vi "Autonomous.vi"() -> ()   [LabVIEW 2023]
doc: "This VI starts when autonomous period begins, and will automatically be terminated when it ends. You can carry out timed or sensor driven operations directly to I/O or to subsystems without needing to return to the caller."
uses:
  <vilib>/Rock Robotics/WPI/Framework/Command Status Info.ctl
  <vilib>/Rock Robotics/WPI/Framework/Completion Status.ctl
  <vilib>/Rock Robotics/WPI/Framework/Completion Notifier.ctl
  Drive/Implementation/Drive Operations.ctl
  Support Code/Teleop Util/Coral States.ctl
  Support Code/Teleop Util/Scoring Levels.ctl
  Coral/Implementation/Coral Operations.ctl
  <vilib>/Rock Robotics/WPI/Utilities/WPI_GetSetVariantRefNum.vi
  Framework/Robot Global Data.vi
  <vilib>/Rock Robotics/Network Tables/NT Read String.vi
  <vilib>/Rock Robotics/Network Tables/NT Read String Array.vi
  <vilib>/Utility/file.llb/Read Delimited Spreadsheet (string).vi
panel:
  in  "Command Info Out 4":T1
  in  "Is Blue Alliance? 5":bool=TRUE
  in  "Command Info Out 3":T1
  in  "Is Blue Alliance? 4":bool=TRUE
  in  "Command Info Out 2":T1
  in  "Is Blue Alliance? 3":bool=TRUE
  in  "Command Info Out":T1
  in  "Is Blue Alliance? 2":bool=TRUE
  in  "Is Blue Alliance?":bool=TRUE
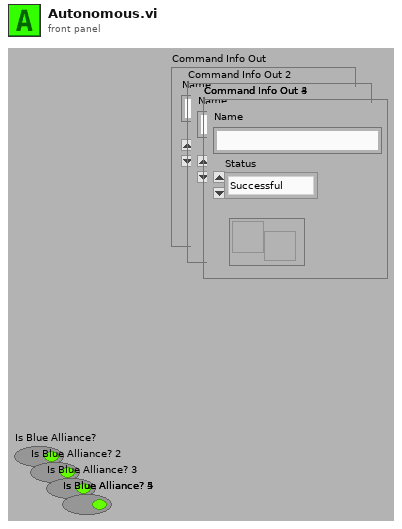
[diagram p1: front panel]
types:
  T1 = typedef "Command Status Info.ctl" = cluster{"Name":string, "Status":T2, "notifier out":T3}
  T2 = typedef "Completion Status.ctl" = enum16{"Successful", "Aborted", "Incomplete"}
  T3 = typedef "Completion Notifier.ctl" = refnum<notifier>
  T4 = typedef "WPI_JoystickDevRef.ctl" = cluster{"Device":T5}
  T5 = typedef "WPI_JoystickDeviceEnum.ctl" = enum16{"USB 0", "USB 1", "USB 2", "USB 3", "USB 4", "USB 5"}
  T6 = typedef "Drive Operations.ctl" = enum16{"Reserve", "Read Current", "Immediate", "Calibrate", "Reef Align", "Auto", "Old Reef Align"}
  T7 = typedef "Coral Operations.ctl" = enum16{"Reserve", "Read Current", "Immediate", "Calibrate"}
  T8 = typedef "Scoring Levels.ctl" = enum16{"Trough", "L2", "L3", "L4", "Default"}
  T9 = typedef "Coral States.ctl" = enum16{"Grounded", "Coral Intake", "Scoring Sequence", "Hold Position", "Score", "Manual Override", "Climb Safety Mode"}
  T10 = cluster{dbl, "Command out":cluster{"Name":string, "vi reference":refnum<vi>, i32[], variant[]}}[]
  T11 = typedef "Robot Velocities.ctl" = cluster{"X Velocity":dbl, "Y Velocity":dbl, "Rotational \nVelocity":dbl}
  T12 = typedef "CTRE_PigeonIMU_DeviceRef.ctl" = cluster{"DeviceStatus":errorcluster, "Device Number":u8, "Type":T13, "Device ID":u32, "Handle":u64, "UsageFrame":u32, "Library Path":path}
  T13 = typedef "CTRE_PigeonIMU_ConnectionType.ctl" = u32
  T14 = cluster{"Velocities":T11[], "Positions":cluster{"x":dbl, "y":dbl, "th":dbl}[], cluster{dbl, "Command out":cluster{"Name":string, "vi reference":refnum<vi>, i32[], variant[]}}[], "Zero Velocity?":bool[]}
  T15 = cluster{"Trough":dbl, "L2":dbl, "L3":dbl, "L4":dbl}
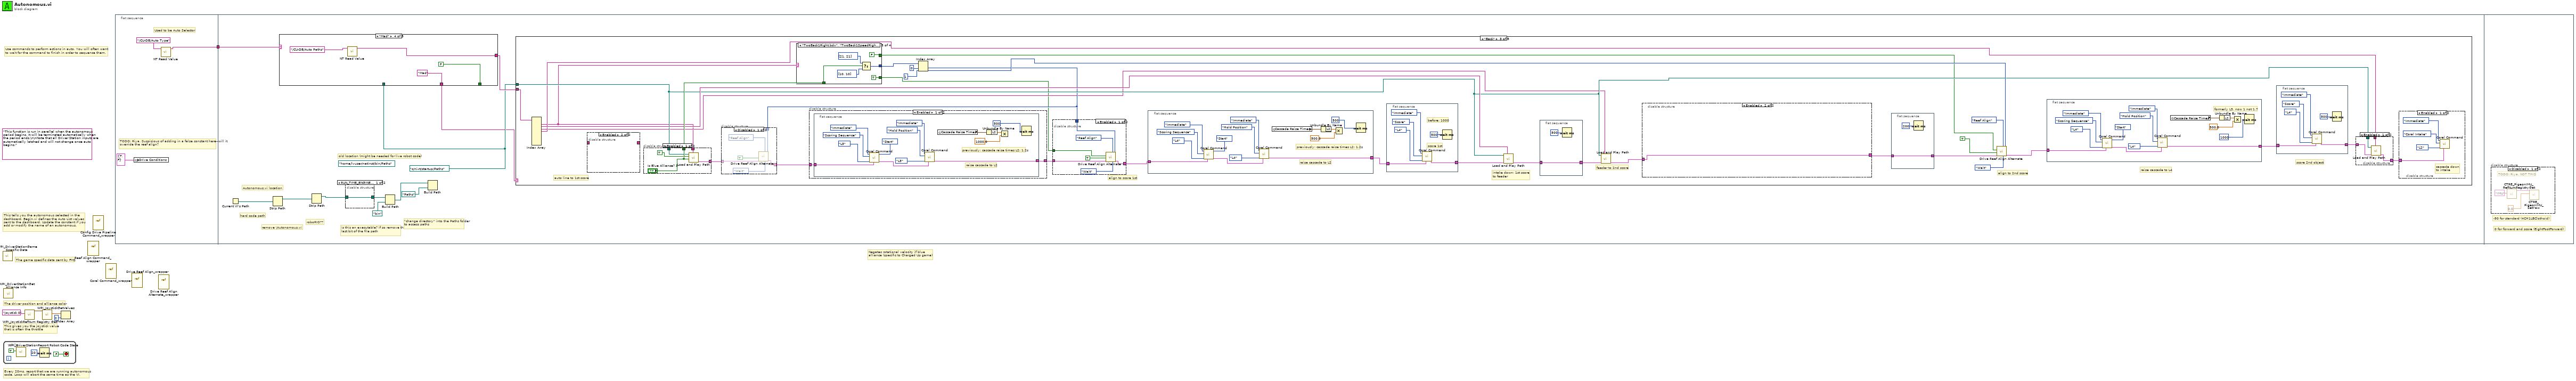
[diagram p0: block diagram]
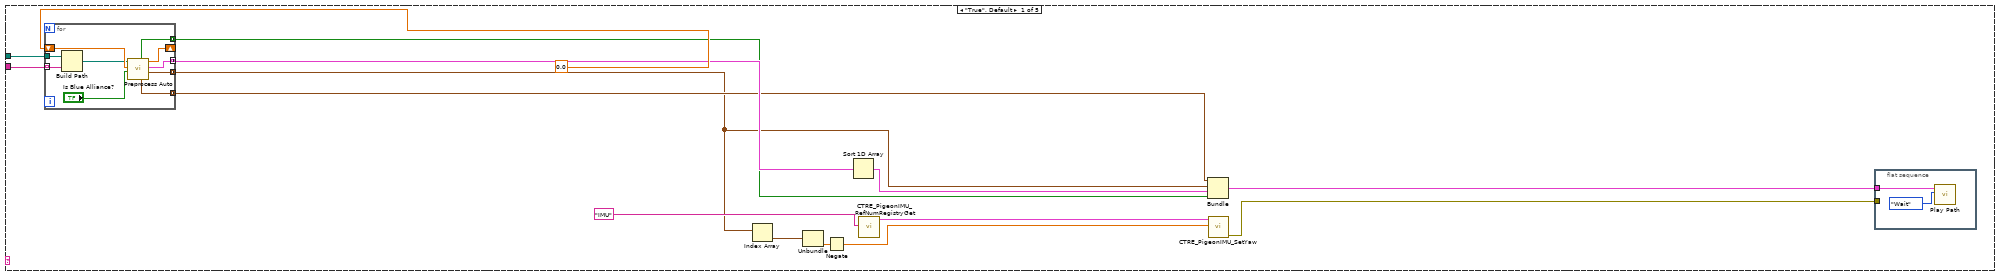
[diagram p2: hidden frame]
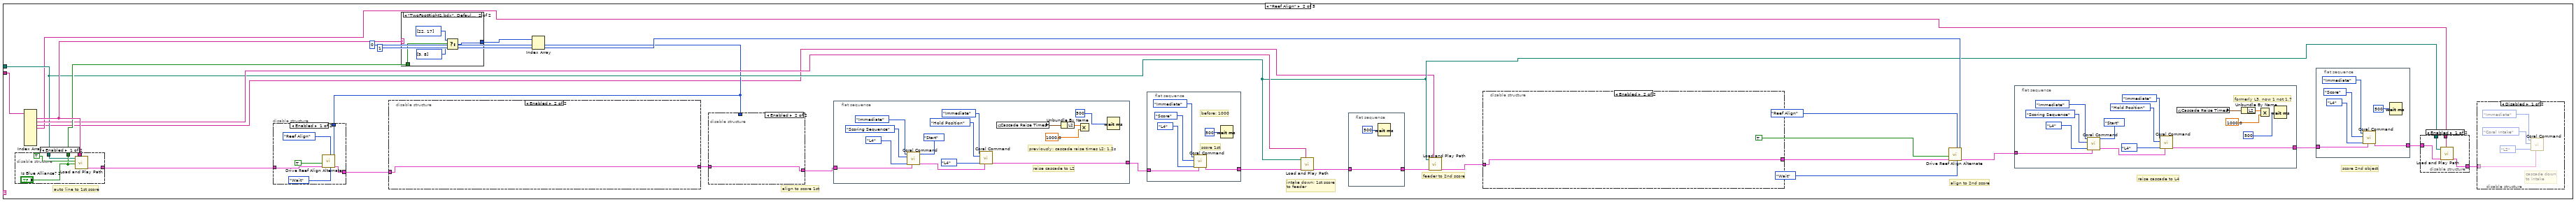
[diagram p3: hidden frame]
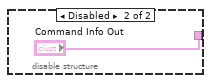
[diagram p4: hidden frame]
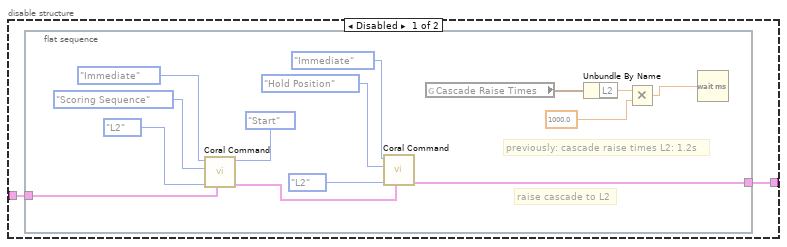
[diagram p6: hidden frame]
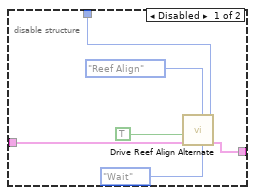
[diagram p8: hidden frame]
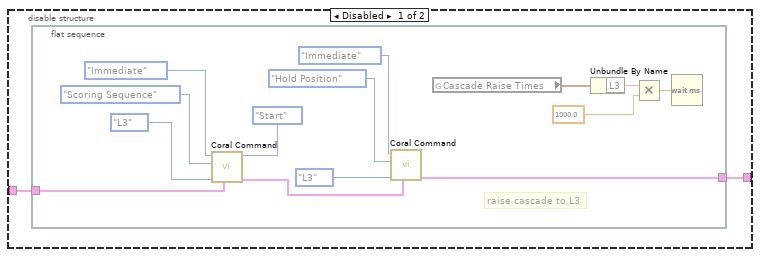
[diagram p9: hidden frame]
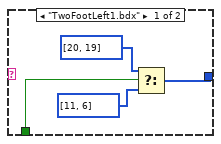
[diagram p11: hidden frame]
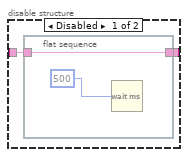
[diagram p12: hidden frame]
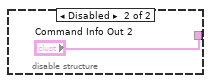
[diagram p13: hidden frame]
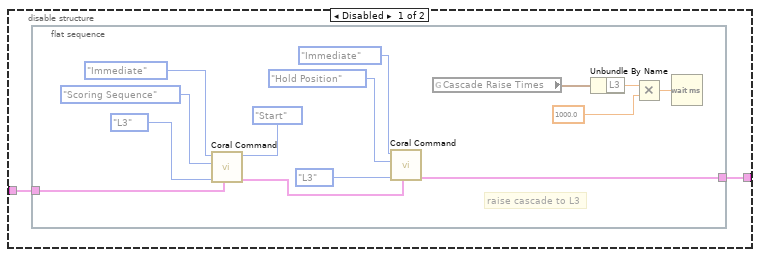
[diagram p18: hidden frame]
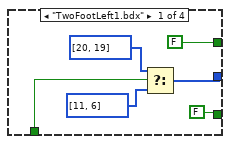
[diagram p20: hidden frame]
diagram:
  (unwired) "This function is run in parallel when the autonomous period begins. It will be terminated automatically when the period ends.\n\nNote that all Driver Station inputs are automatically latched and will not change once auto begins."
  # "Negates rotational velocity if blue alliance (specific to Charged Up game)"
  # "The game specific data sent by FMS"
  # "This tells you the autonomous selected in the \ndashboard. Begin.vi defines the Auto List values\nsent to the dashboard. Update the constant if you\nadd or modify the name of an autonomous."
  # "Every 20ms, report that we are running autonomous\ncode. Loop will abort the same time as the VI."
  # "This gives you the joystick value\nthat is often the throttle"
  # "Use commands to perform actions in auto. You will often want\nto wait for the command to finish in order to sequence them."
  # "The driver position and alliance color"
  n1 = call <vilib>:"WPI_DriverStationGame Specific Data.vi"() -> ()  [unwired: 11 in, 1 out]
  n2 = while {
    stop <- FALSE stop-if-true
    n3 = call <vilib>:"WPI_DriverStationReport Robot Code State.vi"("Autonomous"=TRUE) -> ()  [unwired: 10 in, 1 out]
    n4 = Wait (ms)(milliseconds to wait=u32 20) -> ()  [unwired: 1 out]
  }
  n5 = call <vilib>:"WPI_DriverStationGet Alliance Info.vi"() -> ()  [unwired: 12 out]
  n6 = call <vilib>:"WPI_JoystickRefNum Registry Get.vi"("refnum name"="Joystick 0") -> ("JoystickDevRef"=w4:T4)  [unwired: 1 in, 9 out]
  n7 = call <vilib>:"WPI_JoystickGetValues.vi"("JoystickDevRef"=w4) -> ("Axes"=w3:dbl[])  [unwired: 6 in, 4 out]
  n8 = Index Array(array=w3, index=2) -> ()  [unwired: 1 out]
  n9 = vi-ref "Reef Align Command_wrapper.vi"() -> ()  [unwired: 1 out]
  n10 = vi-ref "Config Drive Pipeline Command_wrapper.vi"() -> ()  [unwired: 1 out]
  n11 = vi-ref "Coral Command_wrapper.vi"() -> ()  [unwired: 1 out]
  n12 = flat-sequence {
    tunnel: [w9] -> w1
    tunnel: w1 -> [w13]
    frame #0 {
      # "Used to be Auto Selector"
      # "TODO: Riya. Suspicious of adding in a false constant here--will it override the reef align?"
      n13 = global write "Robot Global Data.vi" "Drive Conditions"(cluster{"Field Centric":bool, bool} {"Field Centric"=TRUE, FALSE} ("Drive Conditions")) -> ()
      n14 = call-poly <vilib>:"NT Read Value.vi"("name"="/CU-DB/Auto Type") -> ("value"=w9:string)  [unwired: 8 in, 2 out]
    }
    frame #1 {
      (unwired) path "/home/lvuser/natinst/bin/Paths"
      w14 = path "c:/ni-rt/startup/Paths"
      # "old location (might be needed for live robot code)"
      # "\"change directory\" into the Paths folder to access paths"
      # "is this an executable? if so remove that last bit of the file path"
      # "roboRIO??"
      # "remove \\Autonomous.vi"
      # "Autonomous.vi location"
      # "hard code path"
      n15 = Current VI's Path() -> (path=w19:path)
      n16 = Strip Path(path=w19) -> (stripped path=w20:path)  [unwired: 1 out]
      n17 = case shown="\"Mad\"" w13 {
        tunnel: w14 -> [_ _ _ _ w653]
        tunnel: [w631 w635 w639 w643 w647] -> w17
        tunnel: [TRUE FALSE FALSE FALSE TRUE ("Boolean")] -> _
        tunnel: ["" ("String") "Reef Align" "Back" "Mad" "" ("String")] -> w12
        frame "Manual", Default {
          n18 = call-poly <vilib>:"NT Read Value.vi"("name"="/CU-DB/Auto Paths") -> ("value"=w631:string[])  [unwired: 8 in, 2 out]
        }
        frame "Reef Align" {
          n19 = call-poly <vilib>:"NT Read Value.vi"("name"="/CU-DB/Auto Paths") -> ("value"=w635:string[])  [unwired: 8 in, 2 out]
        }
        frame "Back" {
          n20 = call-poly <vilib>:"NT Read Value.vi"("name"="/CU-DB/Auto Paths") -> ("value"=w639:string[])  [unwired: 8 in, 2 out]
        }
        frame "Mad" {
          n21 = call-poly <vilib>:"NT Read Value.vi"("name"="/CU-DB/Auto Paths") -> ("value"=w643:string[])  [unwired: 8 in, 2 out]
        }
        frame "Aquitaine" {
          n22 = call-poly <vilib>:"NT Read Value.vi"("name"="/CU-DB/Aquitaine") -> ("value"=w654:string)  [unwired: 8 in, 2 out]
          n23 = Build Path(base path=w653, name or relative path=w654) -> (appended path=w652:path)
          n24 = call-poly <vilib>:"Read Delimited Spreadsheet.vi"("file path (dialog if empty)"=w652) -> ("all rows"=w648:string[][])  [unwired: 9 in, 5 out]
          n25 = Array Size(array=w648) -> (size(s)=w651:i32[])
          n26 = Index Array(array=w651, index=0) -> (element=w649:i32)
          n27 = Reshape Array(w648, w649) -> (w647:string[])
        }
      }
      n28 = Strip Path(path=w20) -> (stripped path=w22:path)  [unwired: 1 out]
      n29 = disable-structure shown="RUN_TIME_ENGINE==False" {
        disable-tunnel: [w626 w627] -> w21
        disable-tunnel: w22 -> [w626 w628]
        frame condition #0 (active) {
        }
        frame condition #1 {
          n30 = Strip Path(path=w628) -> (stripped path=w627:path)  [unwired: 1 out]
        }
      }
      n31 = Build Path(base path=w21, name or relative path=path "bin") -> (appended path=w15:path)
      n32 = Build Path(base path=w15, name or relative path=path "Paths") -> ()  [unwired: 1 out]
      n33 = case shown="\"Back\"" w12 {
        tunnel: w17 -> [w26 w78 w223 w391 w539]
        tunnel: w14 -> [w25 w60 w207 w374 w531]
        frame "True", Default {
          n34 = for {
            tunnel: [w44] -> w28 mode=concatenating
            tunnel: [w45] -> w27 mode=concatenating
            shift-right: [w49] -> _
            shift-left: 0.0 -> [w47]
            tunnel: [w48] -> w34 mode=concatenating
            tunnel: [w43] -> w29 mode=concatenating
            tunnel: w25 -> [w40]
            tunnel: w26 -> [w41] mode=indexing
            n35 = Build Path(base path=w40, name or relative path=w41) -> (appended path=w42:path)
            n36 = call "Preprocess Auto.vi"("Is Blue Alliance?"="Is Blue Alliance?", "Start Time"=w47, "appended path"=w42) -> ("Positions"=w45:cluster{"x":dbl, "y":dbl, "th":dbl}[], "Array"=w48:T10, "Finish Time"=w49:dbl, "Velocities"=w44:T11[], "Zero Velocity?"=w43:bool[])  [unwired: 4 in]
          }
          n37 = Index Array(array=w27) -> (element=w33:cluster{"x":dbl, "y":dbl, "th":dbl})  [unwired: 1 in]
          n38 = Unbundle(w33) -> ("th"=w32:dbl)  [unwired: 2 out]
          n39 = Negate(x=w32) -> (-x=w31:dbl)
          n40 = Sort 1D Array(array=w34) -> (sorted array=w30:T10)
          n41 = call <vilib>:"CTRE_PigeonIMU_RefNumRegistryGet.vi"("refnum name"="IMU") -> ("PigeonIMUDevRef"=w37:T12)  [unwired: 9 in, 1 out]
          n42 = Bundle("Velocities"=w28, "Positions"=w27, w30, "Zero Velocity?"=w29) -> (w24:T14)  [unwired: 1 in]
          n43 = call <vilib>:"CTRE_PigeonIMU_SetYaw.vi"("Value"=w31, "PigeonIMUDevRef"=w37) -> ("error out"=w23:errorcluster)  [unwired: 8 in, 1 out]
          n44 = flat-sequence {
            tunnel: w24 -> [w38]
            tunnel: w23 -> [_]
            frame #0 {
              n45 = call "Play Path.vi"("Synchronization"=enum16{"Start", "Wait"}."Wait", "Auto Data"=w38) -> ()  [unwired: 9 in, 1 out]
            }
          }
        }
        frame "Reef Align" {
          # "score 2nd object"
          # "raise cascade to L4"
          # "align to 2nd score"
          # "feeder to 2nd score"
          # "intake down; 1st score\nto feeder"
          # "align to score 1st"
          # "auto line to 1st score"
          n46 = Index Array(array=w78) -> (element #1=w76:string, element #2=w72:string, element #3=w52:string, element #4=w59:string)  [unwired: 9 in, 5 out]
          n47 = disable-structure shown="Enabled" {
            disable-tunnel: w76 -> [w82 _]
            disable-tunnel: ["Is Blue Alliance? 2" _] -> w75
            disable-tunnel: w60 -> [w80 _]
            disable-tunnel: [w79 "Command Info Out"] -> w55
            frame Enabled {
              n48 = call "Load and Play Path.vi"("filename"=w82, "Is Blue Alliance? in"="Is Blue Alliance? 2", "Set IMU?"=TRUE, "Path"=w80) -> ("Command Info Out"=w79:T1)  [unwired: 6 in]
            }
            frame Disabled {
            }
          }
          n49 = case shown="\"TwoFootRight1.bdx\", Default" w76 {
            tunnel: w75 -> [w185 w189]
            tunnel: [w186 w188] -> w74
            frame "TwoFootLeft1.bdx" {
              n50 = Select(t=i32[] [20, 19], s=w185, f=i32[] [11, 6]) -> (s? t:f=w186:i32[])
            }
            frame "TwoFootRight1.bdx", Default {
              n51 = Select(t=i32[] [22, 17], s=w189, f=i32[] [9, 8]) -> (s? t:f=w188:i32[])
            }
          }
          n52 = Index Array(array=w74, index #1=0 ("index"), index #2=1 ("index")) -> (element #1=w53:i32, element #2=w63:i32)
          n53 = disable-structure shown="Enabled" {
            disable-tunnel: w55 -> [w122 w126]
            disable-tunnel: [w121 w126] -> w54
            disable-tunnel: w53 -> [w120 _]
            frame Enabled {
              n54 = call "Drive Reef Align Alternate.vi"("Tag ID"=w120, "Synchronication"=enum16{"Start", "Wait"}."Wait", "Operation"=Drive_Operations."Reef Align", "Command Info In"=w122, "Angle Align"=TRUE) -> ("Command Info Out"=w121:T1)  [unwired: 6 in]
            }
            frame Disabled {
            }
          }
          n55 = disable-structure shown="Enabled" {
            disable-tunnel: [w104 w119] -> w77
            disable-tunnel: w54 -> [w103 w119]
            frame Disabled {
              n56 = flat-sequence {
                tunnel: w103 -> [w118]
                tunnel: [w115] -> w104
                frame #0 {
                  # "previously: cascade raise times L2: 1.2s"
                  # "raise cascade to L2"
                  n57 = call "Coral Command.vi"("Synchronization"=enum16{"Start", "Wait"}."Start", "Command Info In"=w118, "Setpoint State"=Scoring_Levels."L2", "Coral States"=Coral_States."Scoring Sequence", "Operation"=Coral_Operations."Immediate") -> ("Command Info Out"=w116:T1)  [unwired: 5 in]
                  n58 = call "Coral Command.vi"("Command Info In"=w116, "Setpoint State"=Scoring_Levels."L2", "Coral States"=Coral_States."Hold Position", "Operation"=Coral_Operations."Immediate") -> ("Command Info Out"=w115:T1)  [unwired: 6 in]
                  n59 = global read "Robot Global Data.vi" "Cascade Raise Times"() -> (w108:T15)
                  n60 = Unbundle By Name(w108) -> ("L2"=w107:dbl)
                  n61 = Multiply(x=w107, y=1000.0) -> (x*y=w106:dbl)
                  n62 = Wait (ms)(milliseconds to wait=w106) -> ()  [unwired: 1 out]
                }
              }
            }
            frame Enabled {
            }
          }
          n63 = disable-structure shown="Enabled" {
            disable-tunnel: w77 -> [w132 w133]
            disable-tunnel: [w128 w133] -> w51
            disable-tunnel: w53 -> [w127 _]
            frame Disabled {
              n64 = call "Drive Reef Align Alternate.vi"("Tag ID"=w127, "Synchronication"=enum16{"Start", "Wait"}."Wait", "Operation"=Drive_Operations."Reef Align", "Command Info In"=w132, "Angle Align"=TRUE) -> ("Command Info Out"=w128:T1)  [unwired: 6 in]
            }
            frame Enabled {
            }
          }
          n65 = flat-sequence {
            tunnel: w51 -> [w102]
            tunnel: [w99] -> w50
            frame #0 {
              # "previously: cascade raise times L2: 1.2s"
              # "raise cascade to L2"
              n66 = call "Coral Command.vi"("Synchronization"=enum16{"Start", "Wait"}."Start", "Command Info In"=w102, "Setpoint State"=Scoring_Levels."L4", "Coral States"=Coral_States."Scoring Sequence", "Operation"=Coral_Operations."Immediate") -> ("Command Info Out"=w100:T1)  [unwired: 5 in]
              n67 = call "Coral Command.vi"("Command Info In"=w100, "Setpoint State"=Scoring_Levels."L4", "Coral States"=Coral_States."Hold Position", "Operation"=Coral_Operations."Immediate") -> ("Command Info Out"=w99:T1)  [unwired: 6 in]
              n68 = global read "Robot Global Data.vi" "Cascade Raise Times"() -> (w92:T15)
              n69 = Unbundle By Name(w92) -> ("L2"=w91:dbl)
              n70 = Multiply(x=w91, y=1000.0) -> ()  [unwired: 1 out]
              n71 = Wait (ms)(milliseconds to wait=u32 500) -> ()  [unwired: 1 out]
            }
          }
          n72 = flat-sequence {
            tunnel: w50 -> [w183]
            tunnel: [w178] -> w71
            frame #0 {
              # "before: 1000"
              # "score 1st"
              n73 = call "Coral Command.vi"("Command Info In"=w183, "Setpoint State"=Scoring_Levels."L4", "Coral States"=Coral_States."Score", "Operation"=Coral_Operations."Immediate") -> ("Command Info Out"=w178:T1)  [unwired: 6 in]
              n74 = Wait (ms)(milliseconds to wait=u32 500) -> ()  [unwired: 1 out]
            }
          }
          n75 = call "Load and Play Path.vi"("filename"=w72, "Command Info In"=w71, "Path"=w60) -> ("Command Info Out"=w70:T1)  [unwired: 7 in]
          n76 = flat-sequence {
            tunnel: w70 -> [w176]
            tunnel: [w176] -> w69
            frame #0 {
              n77 = Wait (ms)(milliseconds to wait=u32 500) -> ()  [unwired: 1 out]
            }
          }
          n78 = call "Load and Play Path.vi"("filename"=w52, "Command Info In"=w69, "Path"=w60) -> ("Command Info Out"=w68:T1)  [unwired: 7 in]
          n79 = disable-structure shown="Enabled" {
            disable-tunnel: w68 -> [w135 w150]
            disable-tunnel: [w134 w150] -> w66
            frame Disabled {
              n80 = flat-sequence {
                tunnel: w135 -> [w149]
                tunnel: [w146] -> w134
                frame #0 {
                  # "raise cascade to L3"
                  n81 = call "Coral Command.vi"("Synchronization"=enum16{"Start", "Wait"}."Start", "Command Info In"=w149, "Setpoint State"=Scoring_Levels."L3", "Coral States"=Coral_States."Scoring Sequence", "Operation"=Coral_Operations."Immediate") -> ("Command Info Out"=w147:T1)  [unwired: 5 in]
                  n82 = call "Coral Command.vi"("Command Info In"=w147, "Setpoint State"=Scoring_Levels."L3", "Coral States"=Coral_States."Hold Position", "Operation"=Coral_Operations."Immediate") -> ("Command Info Out"=w146:T1)  [unwired: 6 in]
                  n83 = global read "Robot Global Data.vi" "Cascade Raise Times"() -> (w139:T15)
                  n84 = Unbundle By Name(w139) -> ("L3"=w138:dbl)
                  n85 = Multiply(x=w138, y=1000.0) -> (x*y=w137:dbl)
                  n86 = Wait (ms)(milliseconds to wait=w137) -> ()  [unwired: 1 out]
                }
              }
            }
            frame Enabled {
            }
          }
          n87 = call "Drive Reef Align Alternate.vi"("Tag ID"=w63, "Synchronication"=enum16{"Start", "Wait"}."Wait", "Operation"=Drive_Operations."Reef Align", "Command Info In"=w66, "Angle Align"=TRUE) -> ("Command Info Out"=w57:T1)  [unwired: 6 in]
          n88 = flat-sequence {
            tunnel: w57 -> [w164]
            tunnel: [w161] -> w56
            frame #0 {
              # "formerly L3, now 1 not 1.7"
              n89 = call "Coral Command.vi"("Synchronization"=enum16{"Start", "Wait"}."Start", "Command Info In"=w164, "Setpoint State"=Scoring_Levels."L4", "Coral States"=Coral_States."Scoring Sequence", "Operation"=Coral_Operations."Immediate") -> ("Command Info Out"=w162:T1)  [unwired: 5 in]
              n90 = call "Coral Command.vi"("Command Info In"=w162, "Setpoint State"=Scoring_Levels."L4", "Coral States"=Coral_States."Hold Position", "Operation"=Coral_Operations."Immediate") -> ("Command Info Out"=w161:T1)  [unwired: 6 in]
              n91 = global read "Robot Global Data.vi" "Cascade Raise Times"() -> (w154:T15)
              n92 = Unbundle By Name(w154) -> ("L2"=w153:dbl)
              n93 = Multiply(x=w153, y=1000.0) -> ()  [unwired: 1 out]
              n94 = Wait (ms)(milliseconds to wait=u32 500) -> ()  [unwired: 1 out]
            }
          }
          n95 = flat-sequence {
            tunnel: w56 -> [w175]
            tunnel: [w170] -> w61
            frame #0 {
              n96 = call "Coral Command.vi"("Command Info In"=w175, "Setpoint State"=Scoring_Levels."L4", "Coral States"=Coral_States."Score", "Operation"=Coral_Operations."Immediate") -> ("Command Info Out"=w170:T1)  [unwired: 6 in]
              n97 = Wait (ms)(milliseconds to wait=u32 500) -> ()  [unwired: 1 out]
            }
          }
          n98 = disable-structure shown="Enabled" {
            disable-tunnel: w61 -> [w168 w169]
            disable-tunnel: w60 -> [w167 _]
            disable-tunnel: w59 -> [w166 _]
            disable-tunnel: [w165 w169] -> w58
            frame Enabled {
              n99 = call "Load and Play Path.vi"("filename"=w166, "Command Info In"=w168, "Path"=w167) -> ("Command Info Out"=w165:T1)  [unwired: 7 in]
            }
            frame Disabled {
            }
          }
          n100 = disable-structure shown="Disabled" {
            disable-tunnel: w58 -> [w85 _]
            frame Disabled {
              # "cascade down\nto intake"
              n101 = call "Coral Command.vi"("Command Info In"=w85, "Setpoint State"=Scoring_Levels."L2", "Coral States"=Coral_States."Coral Intake", "Operation"=Coral_Operations."Immediate") -> ()  [unwired: 6 in, 1 out]
            }
            frame Enabled {
            }
          }
        }
        frame "Back" {
          # "score 2nd object"
          # "raise cascade to L4"
          # "align to 2nd score"
          # "feeder to 2nd score"
          # "intake down; 1st score\nto feeder"
          # "align to score 1st"
          # "auto line to 1st score"
          n102 = Index Array(array=w223) -> (element #1=w192:string, element #2=w218:string, element #3=w199:string, element #4=w206:string)  [unwired: 9 in, 5 out]
          n103 = disable-structure shown="Enabled" {
            disable-tunnel: _ -> [w225 _]
            disable-tunnel: [w224 _] -> _
            frame Disabled {
              n104 = flat-sequence {
                tunnel: w225 -> [w227]
                tunnel: [w227] -> w224
                frame #0 {
                  n105 = Wait (ms)(milliseconds to wait=u32 500) -> ()  [unwired: 1 out]
                }
              }
            }
            frame Enabled {
            }
          }
          n106 = disable-structure shown="Enabled" {
            disable-tunnel: w192 -> [w233 _]
            disable-tunnel: ["Is Blue Alliance? 3" _] -> w221
            disable-tunnel: w207 -> [w231 _]
            disable-tunnel: [w230 "Command Info Out 2"] -> w202
            frame Enabled {
              n107 = call "Load and Play Path.vi"("filename"=w233, "Is Blue Alliance? in"="Is Blue Alliance? 3", "Set IMU?"=TRUE, "Path"=w231) -> ("Command Info Out"=w230:T1)  [unwired: 6 in]
            }
            frame Disabled {
            }
          }
          n108 = case shown="\"TwoBack1Right.bdx\", \"TwoBack1SpeedRight.bdx\"" w192 {
            tunnel: w221 -> [w339 w345 w351 w357]
            tunnel: [w340 w344 w350 w356] -> w220
            tunnel: [FALSE FALSE TRUE FALSE] -> w194
            tunnel: [FALSE TRUE FALSE FALSE] -> w193
            frame "TwoFootLeft1.bdx" {
              n109 = Select(t=i32[] [20, 19], s=w339, f=i32[] [11, 6]) -> (s? t:f=w340:i32[])
            }
            frame "TwoBack1.bdx", "TwoBack1Speed.bdx", Default {
              n110 = Select(t=i32[] [21, 21], s=w345, f=i32[] [10, 10]) -> (s? t:f=w344:i32[])
            }
            frame "TwoBack1Right.bdx", "TwoBack1SpeedRight.bdx" {
              n111 = Select(t=i32[] [21, 21], s=w351, f=i32[] [10, 10]) -> (s? t:f=w350:i32[])
            }
            frame "TwoFootRight1.bdx" {
              n112 = Select(t=i32[] [22, 17], s=w357, f=i32[] [9, 8]) -> (s? t:f=w356:i32[])
            }
          }
          n113 = Index Array(array=w220, index #1=0 ("index"), index #2=1 ("index")) -> (element #1=w200:i32, element #2=w210:i32)
          n114 = disable-structure shown="Disabled" {
            disable-tunnel: w202 -> [w273 w277]
            disable-tunnel: [w272 w277] -> w201
            disable-tunnel: w200 -> [w271 _]
            frame Disabled {
              n115 = call "Drive Reef Align Alternate.vi"("Tag ID"=w271, "Synchronication"=enum16{"Start", "Wait"}."Wait", "Operation"=Drive_Operations."Reef Align", "Command Info In"=w273, "Angle Align"=TRUE) -> ("Command Info Out"=w272:T1)  [unwired: 6 in]
            }
            frame Enabled {
            }
          }
          n116 = disable-structure shown="Enabled" {
            disable-tunnel: [w255 w270] -> w222
            disable-tunnel: w201 -> [w254 w270]
            frame Enabled {
              n117 = flat-sequence {
                tunnel: w254 -> [w269]
                tunnel: [w266] -> w255
                frame #0 {
                  # "previously: cascade raise times L2: 1.2s"
                  # "raise cascade to L2"
                  n118 = call "Coral Command.vi"("Synchronization"=enum16{"Start", "Wait"}."Start", "Command Info In"=w269, "Setpoint State"=Scoring_Levels."L3", "Coral States"=Coral_States."Scoring Sequence", "Operation"=Coral_Operations."Immediate") -> ("Command Info Out"=w267:T1)  [unwired: 5 in]
                  n119 = call "Coral Command.vi"("Command Info In"=w267, "Setpoint State"=Scoring_Levels."L3", "Coral States"=Coral_States."Hold Position", "Operation"=Coral_Operations."Immediate") -> ("Command Info Out"=w266:T1)  [unwired: 6 in]
                  n120 = global read "Robot Global Data.vi" "Cascade Raise Times"() -> (w259:T15)
                  n121 = Unbundle By Name(w259) -> ("L2"=w258:dbl)
                  n122 = Multiply(x=w258, y=1000.0) -> ()  [unwired: 1 out]
                  n123 = Wait (ms)(milliseconds to wait=u32 500) -> ()  [unwired: 1 out]
                }
              }
            }
            frame Disabled {
            }
          }
          n124 = disable-structure shown="Enabled" {
            disable-tunnel: w222 -> [w284 w285]
            disable-tunnel: [w280 w285] -> w198
            disable-tunnel: w200 -> [w279 _]
            disable-tunnel: w194 -> [w278 _]
            frame Enabled {
              n125 = call "Drive Reef Align Alternate.vi"("Tag ID"=w279, "Synchronication"=enum16{"Start", "Wait"}."Wait", "Operation"=Drive_Operations."Reef Align", "Command Info In"=w284, "Angle Align"=TRUE, "Left side"=w278) -> ("Command Info Out"=w280:T1)  [unwired: 5 in]
            }
            frame Disabled {
            }
          }
          n126 = flat-sequence {
            tunnel: w198 -> [w253]
            tunnel: [w250] -> w197
            frame #0 {
              # "previously: cascade raise times L2: 1.2s"
              # "raise cascade to L2"
              n127 = call "Coral Command.vi"("Synchronization"=enum16{"Start", "Wait"}."Start", "Command Info In"=w253, "Setpoint State"=Scoring_Levels."L4", "Coral States"=Coral_States."Scoring Sequence", "Operation"=Coral_Operations."Immediate") -> ("Command Info Out"=w251:T1)  [unwired: 5 in]
              n128 = call "Coral Command.vi"("Command Info In"=w251, "Setpoint State"=Scoring_Levels."L4", "Coral States"=Coral_States."Hold Position", "Operation"=Coral_Operations."Immediate") -> ("Command Info Out"=w250:T1)  [unwired: 6 in]
              n129 = global read "Robot Global Data.vi" "Cascade Raise Times"() -> (w243:T15)
              n130 = Unbundle By Name(w243) -> ("L2"=w242:dbl)
              n131 = Multiply(x=w242, y=500.0) -> ()  [unwired: 1 out]
              n132 = Wait (ms)(milliseconds to wait=u32 500) -> ()  [unwired: 1 out]
            }
          }
          n133 = flat-sequence {
            tunnel: w197 -> [w335]
            tunnel: [w330] -> w217
            frame #0 {
              # "before: 1000"
              # "score 1st"
              n134 = call "Coral Command.vi"("Command Info In"=w335, "Setpoint State"=Scoring_Levels."L4", "Coral States"=Coral_States."Score", "Operation"=Coral_Operations."Immediate") -> ("Command Info Out"=w330:T1)  [unwired: 6 in]
              n135 = Wait (ms)(milliseconds to wait=u32 500) -> ()  [unwired: 1 out]
            }
          }
          n136 = call "Load and Play Path.vi"("filename"=w218, "Command Info In"=w217, "Path"=w207) -> ("Command Info Out"=w216:T1)  [unwired: 7 in]
          n137 = flat-sequence {
            tunnel: w216 -> [w328]
            tunnel: [w328] -> w215
            frame #0 {
              n138 = Wait (ms)(milliseconds to wait=u32 500) -> ()  [unwired: 1 out]
            }
          }
          n139 = call "Load and Play Path.vi"("filename"=w199, "Command Info In"=w215, "Path"=w207) -> ("Command Info Out"=w214:T1)  [unwired: 7 in]
          n140 = disable-structure shown="Enabled" {
            disable-tunnel: w214 -> [w287 w302]
            disable-tunnel: [w286 w302] -> w196
            frame Disabled {
              n141 = flat-sequence {
                tunnel: w287 -> [w301]
                tunnel: [w298] -> w286
                frame #0 {
                  # "raise cascade to L3"
                  n142 = call "Coral Command.vi"("Synchronization"=enum16{"Start", "Wait"}."Start", "Command Info In"=w301, "Setpoint State"=Scoring_Levels."L3", "Coral States"=Coral_States."Scoring Sequence", "Operation"=Coral_Operations."Immediate") -> ("Command Info Out"=w299:T1)  [unwired: 5 in]
                  n143 = call "Coral Command.vi"("Command Info In"=w299, "Setpoint State"=Scoring_Levels."L3", "Coral States"=Coral_States."Hold Position", "Operation"=Coral_Operations."Immediate") -> ("Command Info Out"=w298:T1)  [unwired: 6 in]
                  n144 = global read "Robot Global Data.vi" "Cascade Raise Times"() -> (w291:T15)
                  n145 = Unbundle By Name(w291) -> ("L3"=w290:dbl)
                  n146 = Multiply(x=w290, y=1000.0) -> (x*y=w289:dbl)
                  n147 = Wait (ms)(milliseconds to wait=w289) -> ()  [unwired: 1 out]
                }
              }
            }
            frame Enabled {
            }
          }
          n148 = flat-sequence {
            tunnel: w196 -> [w228]
            tunnel: [w228] -> w195
            frame #0 {
              n149 = Wait (ms)(milliseconds to wait=u32 200) -> ()  [unwired: 1 out]
            }
          }
          n150 = call "Drive Reef Align Alternate.vi"("Tag ID"=w210, "Synchronication"=enum16{"Start", "Wait"}."Wait", "Operation"=Drive_Operations."Reef Align", "Command Info In"=w195, "Angle Align"=TRUE, "Left side"=w193) -> ("Command Info Out"=w204:T1)  [unwired: 5 in]
          n151 = flat-sequence {
            tunnel: w204 -> [w316]
            tunnel: [w313] -> w203
            frame #0 {
              # "formerly L3, now 1 not 1.7"
              n152 = call "Coral Command.vi"("Synchronization"=enum16{"Start", "Wait"}."Start", "Command Info In"=w316, "Setpoint State"=Scoring_Levels."L4", "Coral States"=Coral_States."Scoring Sequence", "Operation"=Coral_Operations."Immediate") -> ("Command Info Out"=w314:T1)  [unwired: 5 in]
              n153 = call "Coral Command.vi"("Command Info In"=w314, "Setpoint State"=Scoring_Levels."L4", "Coral States"=Coral_States."Hold Position", "Operation"=Coral_Operations."Immediate") -> ("Command Info Out"=w313:T1)  [unwired: 6 in]
              n154 = global read "Robot Global Data.vi" "Cascade Raise Times"() -> (w306:T15)
              n155 = Unbundle By Name(w306) -> ("L2"=w305:dbl)
              n156 = Multiply(x=w305, y=500.0) -> ()  [unwired: 1 out]
              n157 = Wait (ms)(milliseconds to wait=u32 1000) -> ()  [unwired: 1 out]
            }
          }
          n158 = flat-sequence {
            tunnel: w203 -> [w327]
            tunnel: [w322] -> w208
            frame #0 {
              n159 = call "Coral Command.vi"("Command Info In"=w327, "Setpoint State"=Scoring_Levels."L4", "Coral States"=Coral_States."Score", "Operation"=Coral_Operations."Immediate") -> ("Command Info Out"=w322:T1)  [unwired: 6 in]
              n160 = Wait (ms)(milliseconds to wait=u32 500) -> ()  [unwired: 1 out]
            }
          }
          n161 = disable-structure shown="Enabled" {
            disable-tunnel: w208 -> [w320 w321]
            disable-tunnel: w207 -> [w319 _]
            disable-tunnel: w206 -> [w318 _]
            disable-tunnel: [w317 w321] -> w205
            frame Enabled {
              n162 = call "Load and Play Path.vi"("filename"=w318, "Command Info In"=w320, "Path"=w319) -> ("Command Info Out"=w317:T1)  [unwired: 7 in]
            }
            frame Disabled {
            }
          }
          n163 = disable-structure shown="Enabled" {
            disable-tunnel: w205 -> [w236 _]
            frame Enabled {
              # "cascade down\nto intake"
              n164 = call "Coral Command.vi"("Command Info In"=w236, "Setpoint State"=Scoring_Levels."L2", "Coral States"=Coral_States."Coral Intake", "Operation"=Coral_Operations."Immediate") -> ()  [unwired: 6 in, 1 out]
            }
            frame Disabled {
            }
          }
        }
        frame "Mad" {
          # "score 2nd object"
          # "raise cascade to L4"
          # "align to 2nd score"
          # "feeder to 2nd score"
          # "intake down; 1st score\nto feeder"
          # "align to score 1st"
          # "auto line to 1st score"
          n165 = Index Array(array=w391) -> (element #1=w389:string, element #2=w385:string, element #3=w366:string, element #4=w373:string)  [unwired: 9 in, 5 out]
          n166 = disable-structure shown="Enabled" {
            disable-tunnel: w389 -> [w397 _]
            disable-tunnel: ["Is Blue Alliance? 5" _] -> w388
            disable-tunnel: w374 -> [w395 _]
            disable-tunnel: [w394 "Command Info Out 4"] -> w369
            frame Enabled {
              n167 = call "Load and Play Path.vi"("filename"=w397, "Is Blue Alliance? in"="Is Blue Alliance? 5", "Set IMU?"=TRUE, "Path"=w395) -> ("Command Info Out"=w394:T1)  [unwired: 6 in]
            }
            frame Disabled {
            }
          }
          n168 = case shown="\"TwoBack1Right.bdx\", \"TwoBack1SpeedRight.bdx\"" w389 {
            tunnel: w388 -> [w503 w509 w515 w521]
            tunnel: [w504 w508 w514 w520] -> w387
            tunnel: [FALSE FALSE TRUE FALSE] -> w361
            tunnel: [FALSE TRUE FALSE FALSE] -> w360
            frame "TwoFootLeft1.bdx" {
              n169 = Select(t=i32[] [20, 19], s=w503, f=i32[] [11, 6]) -> (s? t:f=w504:i32[])
            }
            frame "TwoBack1.bdx", "TwoBack1Speed.bdx", Default {
              n170 = Select(t=i32[] [21, 19], s=w509, f=i32[] [10, 6]) -> (s? t:f=w508:i32[])
            }
            frame "TwoBack1Right.bdx", "TwoBack1SpeedRight.bdx" {
              n171 = Select(t=i32[] [21, 17], s=w515, f=i32[] [10, 8]) -> (s? t:f=w514:i32[])
            }
            frame "TwoFootRight1.bdx" {
              n172 = Select(t=i32[] [22, 17], s=w521, f=i32[] [9, 8]) -> (s? t:f=w520:i32[])
            }
          }
          n173 = Index Array(array=w387, index #1=0 ("index"), index #2=1 ("index")) -> (element #1=w367:i32, element #2=w377:i32)
          n174 = disable-structure shown="Disabled" {
            disable-tunnel: w369 -> [w437 w441]
            disable-tunnel: [w436 w441] -> w368
            disable-tunnel: w367 -> [w435 _]
            frame Disabled {
              n175 = call "Drive Reef Align Alternate.vi"("Tag ID"=w435, "Synchronication"=enum16{"Start", "Wait"}."Wait", "Operation"=Drive_Operations."Reef Align", "Command Info In"=w437, "Angle Align"=TRUE) -> ("Command Info Out"=w436:T1)  [unwired: 6 in]
            }
            frame Enabled {
            }
          }
          n176 = disable-structure shown="Enabled" {
            disable-tunnel: [w419 w434] -> w390
            disable-tunnel: w368 -> [w418 w434]
            frame Enabled {
              n177 = flat-sequence {
                tunnel: w418 -> [w433]
                tunnel: [w430] -> w419
                frame #0 {
                  # "previously: cascade raise times L2: 1.2s"
                  # "raise cascade to L2"
                  n178 = call "Coral Command.vi"("Synchronization"=enum16{"Start", "Wait"}."Start", "Command Info In"=w433, "Setpoint State"=Scoring_Levels."L3", "Coral States"=Coral_States."Scoring Sequence", "Operation"=Coral_Operations."Immediate") -> ("Command Info Out"=w431:T1)  [unwired: 5 in]
                  n179 = call "Coral Command.vi"("Command Info In"=w431, "Setpoint State"=Scoring_Levels."L3", "Coral States"=Coral_States."Hold Position", "Operation"=Coral_Operations."Immediate") -> ("Command Info Out"=w430:T1)  [unwired: 6 in]
                  n180 = global read "Robot Global Data.vi" "Cascade Raise Times"() -> (w423:T15)
                  n181 = Unbundle By Name(w423) -> ("L2"=w422:dbl)
                  n182 = Multiply(x=w422, y=1000.0) -> ()  [unwired: 1 out]
                  n183 = Wait (ms)(milliseconds to wait=u32 500) -> ()  [unwired: 1 out]
                }
              }
            }
            frame Disabled {
            }
          }
          n184 = disable-structure shown="Enabled" {
            disable-tunnel: w390 -> [w448 w449]
            disable-tunnel: [w444 w449] -> w365
            disable-tunnel: w367 -> [w443 _]
            disable-tunnel: w361 -> [w442 _]
            frame Enabled {
              n185 = call "Drive Reef Align Alternate.vi"("Tag ID"=w443, "Synchronication"=enum16{"Start", "Wait"}."Wait", "Operation"=Drive_Operations."Reef Align", "Command Info In"=w448, "Angle Align"=TRUE, "Left side"=w442) -> ("Command Info Out"=w444:T1)  [unwired: 5 in]
            }
            frame Disabled {
            }
          }
          n186 = flat-sequence {
            tunnel: w365 -> [w417]
            tunnel: [w414] -> w364
            frame #0 {
              # "previously: cascade raise times L2: 1.2s"
              # "raise cascade to L2"
              n187 = call "Coral Command.vi"("Synchronization"=enum16{"Start", "Wait"}."Start", "Command Info In"=w417, "Setpoint State"=Scoring_Levels."L4", "Coral States"=Coral_States."Scoring Sequence", "Operation"=Coral_Operations."Immediate") -> ("Command Info Out"=w415:T1)  [unwired: 5 in]
              n188 = call "Coral Command.vi"("Command Info In"=w415, "Setpoint State"=Scoring_Levels."L4", "Coral States"=Coral_States."Hold Position", "Operation"=Coral_Operations."Immediate") -> ("Command Info Out"=w414:T1)  [unwired: 6 in]
              n189 = global read "Robot Global Data.vi" "Cascade Raise Times"() -> (w407:T15)
              n190 = Unbundle By Name(w407) -> ("L2"=w406:dbl)
              n191 = Multiply(x=w406, y=500.0) -> ()  [unwired: 1 out]
              n192 = Wait (ms)(milliseconds to wait=u32 500) -> ()  [unwired: 1 out]
            }
          }
          n193 = flat-sequence {
            tunnel: w364 -> [w499]
            tunnel: [w494] -> w384
            frame #0 {
              # "before: 1000"
              # "score 1st"
              n194 = call "Coral Command.vi"("Command Info In"=w499, "Setpoint State"=Scoring_Levels."L4", "Coral States"=Coral_States."Score", "Operation"=Coral_Operations."Immediate") -> ("Command Info Out"=w494:T1)  [unwired: 6 in]
              n195 = Wait (ms)(milliseconds to wait=u32 500) -> ()  [unwired: 1 out]
            }
          }
          n196 = call "Load and Play Path.vi"("filename"=w385, "Command Info In"=w384, "Path"=w374) -> ("Command Info Out"=w383:T1)  [unwired: 7 in]
          n197 = flat-sequence {
            tunnel: w383 -> [w492]
            tunnel: [w492] -> w382
            frame #0 {
              n198 = Wait (ms)(milliseconds to wait=u32 500) -> ()  [unwired: 1 out]
            }
          }
          n199 = call "Load and Play Path.vi"("filename"=w366, "Command Info In"=w382, "Path"=w374) -> ("Command Info Out"=w381:T1)  [unwired: 7 in]
          n200 = disable-structure shown="Enabled" {
            disable-tunnel: w381 -> [w451 w466]
            disable-tunnel: [w450 w466] -> w363
            frame Disabled {
              n201 = flat-sequence {
                tunnel: w451 -> [w465]
                tunnel: [w462] -> w450
                frame #0 {
                  # "raise cascade to L3"
                  n202 = call "Coral Command.vi"("Synchronization"=enum16{"Start", "Wait"}."Start", "Command Info In"=w465, "Setpoint State"=Scoring_Levels."L3", "Coral States"=Coral_States."Scoring Sequence", "Operation"=Coral_Operations."Immediate") -> ("Command Info Out"=w463:T1)  [unwired: 5 in]
                  n203 = call "Coral Command.vi"("Command Info In"=w463, "Setpoint State"=Scoring_Levels."L3", "Coral States"=Coral_States."Hold Position", "Operation"=Coral_Operations."Immediate") -> ("Command Info Out"=w462:T1)  [unwired: 6 in]
                  n204 = global read "Robot Global Data.vi" "Cascade Raise Times"() -> (w455:T15)
                  n205 = Unbundle By Name(w455) -> ("L3"=w454:dbl)
                  n206 = Multiply(x=w454, y=1000.0) -> (x*y=w453:dbl)
                  n207 = Wait (ms)(milliseconds to wait=w453) -> ()  [unwired: 1 out]
                }
              }
            }
            frame Enabled {
            }
          }
          n208 = flat-sequence {
            tunnel: w363 -> [w392]
            tunnel: [w392] -> w362
            frame #0 {
              n209 = Wait (ms)(milliseconds to wait=u32 200) -> ()  [unwired: 1 out]
            }
          }
          n210 = call "Drive Reef Align Alternate.vi"("Tag ID"=w377, "Synchronication"=enum16{"Start", "Wait"}."Wait", "Operation"=Drive_Operations."Reef Align", "Command Info In"=w362, "Angle Align"=TRUE, "Left side"=w360) -> ("Command Info Out"=w371:T1)  [unwired: 5 in]
          n211 = flat-sequence {
            tunnel: w371 -> [w480]
            tunnel: [w477] -> w370
            frame #0 {
              # "formerly L3, now 1 not 1.7"
              n212 = call "Coral Command.vi"("Synchronization"=enum16{"Start", "Wait"}."Start", "Command Info In"=w480, "Setpoint State"=Scoring_Levels."L4", "Coral States"=Coral_States."Scoring Sequence", "Operation"=Coral_Operations."Immediate") -> ("Command Info Out"=w478:T1)  [unwired: 5 in]
              n213 = call "Coral Command.vi"("Command Info In"=w478, "Setpoint State"=Scoring_Levels."L4", "Coral States"=Coral_States."Hold Position", "Operation"=Coral_Operations."Immediate") -> ("Command Info Out"=w477:T1)  [unwired: 6 in]
              n214 = global read "Robot Global Data.vi" "Cascade Raise Times"() -> (w470:T15)
              n215 = Unbundle By Name(w470) -> ("L2"=w469:dbl)
              n216 = Multiply(x=w469, y=500.0) -> ()  [unwired: 1 out]
              n217 = Wait (ms)(milliseconds to wait=u32 1000) -> ()  [unwired: 1 out]
            }
          }
          n218 = flat-sequence {
            tunnel: w370 -> [w491]
            tunnel: [w486] -> w375
            frame #0 {
              n219 = call "Coral Command.vi"("Command Info In"=w491, "Setpoint State"=Scoring_Levels."L4", "Coral States"=Coral_States."Score", "Operation"=Coral_Operations."Immediate") -> ("Command Info Out"=w486:T1)  [unwired: 6 in]
              n220 = Wait (ms)(milliseconds to wait=u32 500) -> ()  [unwired: 1 out]
            }
          }
          n221 = disable-structure shown="Enabled" {
            disable-tunnel: w375 -> [w484 w485]
            disable-tunnel: w374 -> [w483 _]
            disable-tunnel: w373 -> [w482 _]
            disable-tunnel: [w481 w485] -> w372
            frame Enabled {
              n222 = call "Load and Play Path.vi"("filename"=w482, "Command Info In"=w484, "Path"=w483) -> ("Command Info Out"=w481:T1)  [unwired: 7 in]
            }
            frame Disabled {
            }
          }
          n223 = disable-structure shown="Enabled" {
            disable-tunnel: w372 -> [w400 _]
            frame Enabled {
              # "cascade down\nto intake"
              n224 = call "Coral Command.vi"("Command Info In"=w400, "Setpoint State"=Scoring_Levels."L2", "Coral States"=Coral_States."Coral Intake", "Operation"=Coral_Operations."Immediate") -> ()  [unwired: 6 in, 1 out]
            }
            frame Disabled {
            }
          }
        }
        frame "Short Back" {
          # "align to score 1st"
          # "auto line to 1st score"
          n225 = Index Array(array=w539) -> (element #1=w537:string, element #2=w533:string)  [unwired: 9 in, 7 out]
          n226 = disable-structure shown="Enabled" {
            disable-tunnel: w537 -> [w547 _]
            disable-tunnel: ["Is Blue Alliance? 4" _] -> w536
            disable-tunnel: w531 -> [w545 _]
            disable-tunnel: [w544 "Command Info Out 3"] -> w530
            frame Enabled {
              n227 = call "Load and Play Path.vi"("filename"=w547, "Is Blue Alliance? in"="Is Blue Alliance? 4", "Set IMU?"=TRUE, "Path"=w545) -> ("Command Info Out"=w544:T1)  [unwired: 6 in]
            }
            frame Disabled {
            }
          }
          n228 = case shown="\"TwoBack1Right.bdx\", \"TwoBack1SpeedRight.bdx\"" w537 {
            tunnel: w536 -> [w605 w611 w617 w623]
            tunnel: [w606 w610 w616 w622] -> w535
            tunnel: [FALSE FALSE TRUE FALSE] -> w525
            tunnel: [FALSE TRUE FALSE FALSE] -> _
            frame "TwoFootLeft1.bdx" {
              n229 = Select(t=i32[] [20, 19], s=w605, f=i32[] [11, 6]) -> (s? t:f=w606:i32[])
            }
            frame "TwoBack1.bdx", "TwoBack1Speed.bdx" {
              n230 = Select(t=i32[] [21, 21], s=w611, f=i32[] [10, 10]) -> (s? t:f=w610:i32[])
            }
            frame "TwoBack1Right.bdx", "TwoBack1SpeedRight.bdx" {
              n231 = Select(t=i32[] [21, 21], s=w617, f=i32[] [10, 10]) -> (s? t:f=w616:i32[])
            }
            frame "TwoFootRight1.bdx", Default {
              n232 = Select(t=i32[] [22, 17], s=w623, f=i32[] [9, 8]) -> (s? t:f=w622:i32[])
            }
          }
          n233 = Index Array(array=w535, index=0) -> (element=w528:i32)
          n234 = disable-structure shown="Disabled" {
            disable-tunnel: w530 -> [w583 w587]
            disable-tunnel: [w582 w587] -> w529
            disable-tunnel: w528 -> [w581 _]
            frame Disabled {
              n235 = call "Drive Reef Align Alternate.vi"("Tag ID"=w581, "Synchronication"=enum16{"Start", "Wait"}."Wait", "Operation"=Drive_Operations."Reef Align", "Command Info In"=w583, "Angle Align"=TRUE) -> ("Command Info Out"=w582:T1)  [unwired: 6 in]
            }
            frame Enabled {
            }
          }
          n236 = disable-structure shown="Enabled" {
            disable-tunnel: [w565 w580] -> w538
            disable-tunnel: w529 -> [w564 w580]
            frame Enabled {
              n237 = flat-sequence {
                tunnel: w564 -> [w579]
                tunnel: [w576] -> w565
                frame #0 {
                  # "previously: cascade raise times L2: 1.2s"
                  # "raise cascade to L2"
                  n238 = call "Coral Command.vi"("Synchronization"=enum16{"Start", "Wait"}."Start", "Command Info In"=w579, "Setpoint State"=Scoring_Levels."L3", "Coral States"=Coral_States."Scoring Sequence", "Operation"=Coral_Operations."Immediate") -> ("Command Info Out"=w577:T1)  [unwired: 5 in]
                  n239 = call "Coral Command.vi"("Command Info In"=w577, "Setpoint State"=Scoring_Levels."L3", "Coral States"=Coral_States."Hold Position", "Operation"=Coral_Operations."Immediate") -> ("Command Info Out"=w576:T1)  [unwired: 6 in]
                  n240 = global read "Robot Global Data.vi" "Cascade Raise Times"() -> (w569:T15)
                  n241 = Unbundle By Name(w569) -> ("L2"=w568:dbl)
                  n242 = Multiply(x=w568, y=1000.0) -> ()  [unwired: 1 out]
                  n243 = Wait (ms)(milliseconds to wait=u32 500) -> ()  [unwired: 1 out]
                }
              }
            }
            frame Disabled {
            }
          }
          n244 = disable-structure shown="Enabled" {
            disable-tunnel: w538 -> [w594 w595]
            disable-tunnel: [w590 w595] -> w527
            disable-tunnel: w528 -> [w589 _]
            disable-tunnel: w525 -> [w588 _]
            frame Enabled {
              n245 = call "Drive Reef Align Alternate.vi"("Tag ID"=w589, "Synchronication"=enum16{"Start", "Wait"}."Wait", "Operation"=Drive_Operations."Reef Align", "Command Info In"=w594, "Angle Align"=TRUE, "Left side"=w588) -> ("Command Info Out"=w590:T1)  [unwired: 5 in]
            }
            frame Disabled {
            }
          }
          n246 = flat-sequence {
            tunnel: w527 -> [w563]
            tunnel: [w560] -> w526
            frame #0 {
              # "previously: cascade raise times L2: 1.2s"
              # "raise cascade to L2"
              n247 = call "Coral Command.vi"("Synchronization"=enum16{"Start", "Wait"}."Start", "Command Info In"=w563, "Setpoint State"=Scoring_Levels."L4", "Coral States"=Coral_States."Scoring Sequence", "Operation"=Coral_Operations."Immediate") -> ("Command Info Out"=w561:T1)  [unwired: 5 in]
              n248 = call "Coral Command.vi"("Command Info In"=w561, "Setpoint State"=Scoring_Levels."L4", "Coral States"=Coral_States."Hold Position", "Operation"=Coral_Operations."Immediate") -> ("Command Info Out"=w560:T1)  [unwired: 6 in]
              n249 = global read "Robot Global Data.vi" "Cascade Raise Times"() -> (w553:T15)
              n250 = Unbundle By Name(w553) -> ("L2"=w552:dbl)
              n251 = Multiply(x=w552, y=500.0) -> ()  [unwired: 1 out]
              n252 = Wait (ms)(milliseconds to wait=u32 500) -> ()  [unwired: 1 out]
            }
          }
          n253 = flat-sequence {
            tunnel: w526 -> [w601]
            tunnel: [w596] -> w532
            frame #0 {
              # "before: 1000"
              # "score 1st"
              n254 = call "Coral Command.vi"("Command Info In"=w601, "Setpoint State"=Scoring_Levels."L4", "Coral States"=Coral_States."Score", "Operation"=Coral_Operations."Immediate") -> ("Command Info Out"=w596:T1)  [unwired: 6 in]
              n255 = Wait (ms)(milliseconds to wait=u32 500) -> ()  [unwired: 1 out]
            }
          }
          n256 = call "Load and Play Path.vi"("filename"=w533, "Command Info In"=w532, "Path"=w531) -> ("Command Info Out"=w524:T1)  [unwired: 7 in]
          n257 = disable-structure shown="Enabled" {
            disable-tunnel: w524 -> [w540 _]
            frame Enabled {
              # "cascade down\nto intake"
              n258 = call "Coral Command.vi"("Command Info In"=w540, "Setpoint State"=Scoring_Levels."L2", "Coral States"=Coral_States."Coral Intake", "Operation"=Coral_Operations."Immediate") -> ()  [unwired: 6 in, 1 out]
            }
            frame Disabled {
            }
          }
        }
      }
    }
    frame #2 {
      # "0 for forward and score (EightFootForward)"
      # "-90 for standard (4CH1LBClothoid)"
      n259 = disable-structure shown="Disabled" {
        frame Disabled {
          # "TODO: Riya. NOT THIS"
          n260 = call <vilib>:"CTRE_PigeonIMU_RefNumRegistryGet.vi"("refnum name"="IMU") -> ("PigeonIMUDevRef"=w656:T12)  [unwired: 9 in, 1 out]
          n261 = call <vilib>:"CTRE_PigeonIMU_SetYaw.vi"("Value"=0.0, "PigeonIMUDevRef"=w656) -> ()  [unwired: 8 in, 2 out]
        }
        frame Enabled {
        }
      }
    }
  }
  n262 = vi-ref "Drive Reef Align_wrapper.vi"() -> ()  [unwired: 1 out]
  n263 = vi-ref "Drive Reef Align Alternate_wrapper.vi"() -> ()  [unwired: 1 out]
